vi "Destroy.vi"(8 "error in (no error)":errorcluster, 11 "SSL-Lib in":refnum<class "SSL-Lib.lvclass">) -> (0 "error out":errorcluster)   [LabVIEW 2013, in "SSL_Lib.lvlib" / "SSL-Lib.lvclass"]
uses:
  SSL-Lib.lvclass
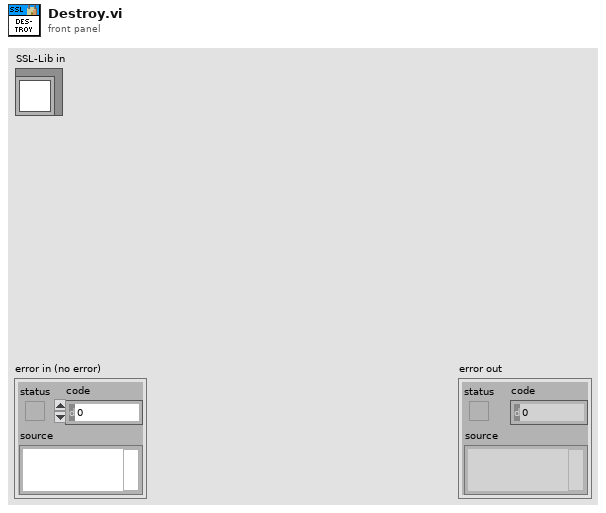
[diagram p1: front panel]
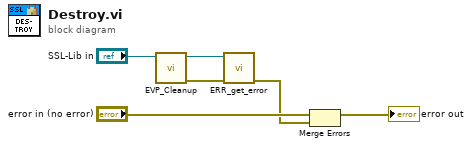
[diagram p0: block diagram]
diagram:
  n1 = call "EVP_Cleanup.vi"("SSL-Lib in"="SSL-Lib in") -> ("error out"=w3:errorcluster, "SSL-Lib out"=w1:refnum<class "SSL-Lib.lvclass">)  [unwired: 9 in]
  n2 = call "ERR_get_error.vi"("error in (no error)"=w3, "SSL-Lib in"=w1) -> ("error out"=w2:errorcluster)  [unwired: 8 in, 1 out]
  n3 = Merge Errors("error in (no error)", w2) -> (→"error out":errorcluster)
